vi "AlliGator Filter Phasors in ROI(s).vi"(7 "Phasor Plot Image":T1, 8 "error in (no error)":errorcluster, 9 "All Phasor Plot ROIs":bool, 10 "Selected Phasor Plot ROI(s)":bool, 11 "Phasor Array in":csg[](array[numeric])) -> (0 "error out":errorcluster, 1 "Message":string, 3 "Phasor Array out":csg[](array[numeric]))   [LabVIEW 2021, in "AlliGator Phasor Plot.lvlib"]
doc: "Returns an array of phasor values located within the selected Phasor Plot ROI (or All ROIs)."
uses:
  AlliGator Phasor Plot.lvlib
  <vilib>/vision/Image Controls.llb/IMAQ Image.ctl
  Globals, Variables, Constants/AlliGator Variables List.ctl
  Phasor Ratio/AlliGator Phasor Plot Reference Points.ctl
  91eb7ac0-7abc-46e1-b76d-bce32f8ebfb4.vi
  <userlib>/_OpenG.lib/array/array.llb/Filter 1D Array (CSG)__ogtk.vi
  ROIs/AlliGator ROIs.lvlib
  <vilib>/vision/NI_Vision_Development_Module.lvlib
  Globals, Variables, Constants/AlliGator Globals, Variables & Constants.lvlib
  Phasor Ratio/AlliGator Phasor Ratio.lvlib
  Strings/Strings.lvlib
  <userlib>/_OpenG.lib/array/array.llb/openg_array.lvlib
  Error/Error.lvlib
panel:
  # "see the AlliGator License on the block diagram (Ctrl+E or Window:Show Block Diagram)"
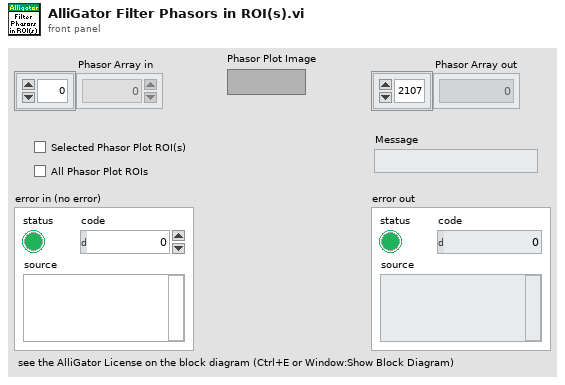
[diagram p1: front panel]
types:
  T1 = typedef "IMAQ Image.ctl" = refnum<image>
  T2 = typedef "AlliGator Phasor Ratio.lvlib/AlliGator Phasor Plot Reference Points.ctl" = cluster{"O_h":dbl, "O_v":dbl, "1_h":dbl, "1_v":dbl}
  T3 = typedef "AlliGator Globals, Variables & Constants.lvlib/AlliGator Variables List.ctl" = enum16{"---- GUI ----", "GUI:Initialization Status", "GUI:State Indicators Refnum", "GUI:Original AlliGator Menu Items", "GUI:Current Action Loop State", "GUI:Script in progress", "GUI:Playback", "GUI:Loop Playback", "GUI:Search ROI Used", "GUI:Search ROI", "Decay Graph Max Legend Size", "Intensity Graph Max Legend Size", "Decay Statistics Graph Max Legend Size", "Phasor Graph Max Legend Size", "Phasor Ratio Graph Max Legend Size", "Lifetime Graph Max Legend Size", "---- Files ----", "Files:Export Dataset Frames as Individual Files", "Files:Show Batch Export Help Balloons", "Files:Frames in Dataset", "Files:ptu File Frame Start Indices", "Files:Current Frame in Dataset", "Files:Current Frame Timestamp", "Files:Dataset Loaded", "Files:Dataset Metadata", "Files:Dataset Channel", "Files:Dataset Data Description", "Files:Background Dataset Metadata", "Files:Background Dataset Channel", "Files:Background Dataset Data Description", "Files:Background File Subtraction", "Files:Background File Path", "Files:Background File Pile-up Correction", "Files:Background File Pixel Well Capacity", "Files:Background File Scaling Factor", "Files:Current Dataset Load Settings", "Files:Dataset Path", "Files:ICCD-specific Information", "Files:Macrotime Gate Separation", "------ Python Plugins ------", "Python Plugins:Information", "Python Plugins:Python Session", "Python Plugins:Valid Python Session?", "---- Source Image ----", "Source Image:ROIs", "Source Image:Current ROI", "Source Image:ROI Event Refnum", "X_Source Image:Display Range", "X_Source Image:Palette Information", "X_Source Image:Type of Displayed Image", "X_Time Gate Slider", "Source Image:Palette List", "Source Image:Scale", "Source Image:ROI Overlay Color", "Source Image:Overlay to Erase", "Source Image:Is Displayed Image Accumulated", "Source Image:White Light Image Modified", "Source Image:Mask Image Modified", "---- Image Profile Window ----", "Image Profile:Window Event Refnum", "Image Profile:IntensityType", "Image Profile:Intensity Average Type", "Image Profile:Intensity-weighted SDV", "Image Profile:Box Profile Type", "Image Profile:Window Open", "Image Profile:Plotted Fit Parameter", "------ Phasor Graph -------", "Phasor Graph:Show Line", "---- Phasor Plot ---", "Phasor Plot:Parameters Changed", "Phasor Plot:FLI Dataset Modified since last Calculation", "Phasor Harmonics Data", "Selected Phasor Harmonics", "Phasor Harmonic Manager Event Refnum", "Phasor Plot:ROIs", "Phasor Plot:Current ROI", "Phasor Plot:ROI Event Refnum", "Phasor Plot:Image Reference Points", "Phasor Plot:Computed", "Phasor Plot:Palette Information", "Phasor Plot:Palette List", "Phasor Plot:Phasor Ratio Palette Information", "Phasor Plot:Phasor Ratio Palette List", "Phasor Plot:Image Scale", "Phasor Plot:Image Overlay to Erase", "Phasor Plot:Image Elements to Update", "Phasor Plot:Current Calculation Parameters", "Phasor Plot:Current Calibration Options", "Phasor Plot:Reset Cumulated Phasor Plot", "Phasor Plot:Reference 1", "Phasor Plot:Lifetime Reference 1", "Phasor Plot:Reference 1 Frequency", "Phasor Plot:Reference 2", "Phasor Plot:Lifetime Reference 2", "Phasor Plot:Reference 2 Frequency", "---- Decay Analysis ----", "Number of Selected Decays to Fit", "LS Fit Results", "LAR Fit Results", "BS Fit Results", "Last Decay Max - Min", "Best Fit Parameters", "Best Fit Parameter Names", "Actual Size X", "Actual Size Y", "Binning X", "Binning Y", "Actual # Gates", "Dataset Number", "Gates to...", "Gates Skipped", "Gates to keep", "Gate Step", "Gate Separation", "Reversed Gates", "Pile-up Correction", "Pixel Well Capacity", "Background Subtracted", "Background Subtraction Method", "Background Definition Range", "Background File (deprecated)", "Number of Dataset Accumulated", "Array of Accumulated Dataset Paths", "Do Averaged Datasets", "Destination File Path", "Process Plot Target", "Use 1/D as Phasor Frequency", "---- Decay Fit Parameter Map -----", "Decay Fit Parameter Map:Palette Information", "Decay Fit Parameter Map:Palette List", "Decay Fit Parameter Map:X Resolution", "Decay Fit Parameter Map:Y Resolution", "---- Parameter Map ----", "Parameter Map:Palette Information", "Parameter Map:Palette List", "------- Local Decay Window ---------", "Local Decay Graph Window:Event Refnum", "Local Decay Graph Window:Use normalized IRF for convolution", "----- Miscellaneous ----", "Misc:Skippable Dialog Windows Status"}
  T4 = typedef "Image Type" = u32
  T5 = typedef "Image.lvlib/Named ROI Description.ctl" = cluster{"ROI Descriptor":T6, "ROI Name":string, "Overlay Color":u32}
  T6 = typedef "ROI Descriptor" = cluster{"Global Rectangle":i32[], "Contours":cluster{"ID":enum32{"External", "Internal"}, "Type":u32, "Coordinates":i32[]}[]}
  T7 = cluster{"Phasor Plot x":dbl, "Phasor Plot y":dbl}
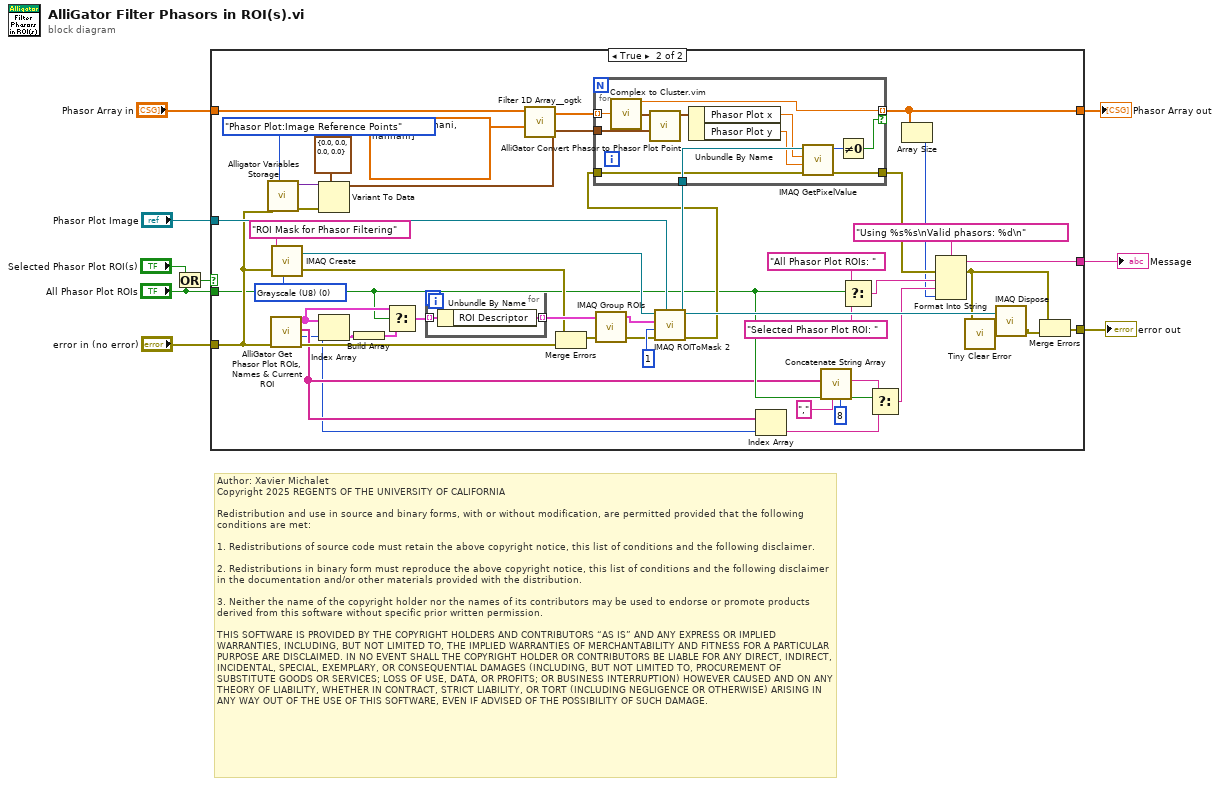
[diagram p0: block diagram]
diagram:
  # "Author: Xavier Michalet\nCopyright 2025 REGENTS OF THE UNIVERSITY OF CALIFORNIA\n\nRedistribution and use in source and binary forms, with or without modification, are permitted provided that the following conditions are met:\n\n1. Redistributions of source code must retain the above copyright notice, this list of conditions and the following disclaimer.\n\n2. Redistributions in binary form must reproduce the above copyright notice, this list of conditions and the following disclaimer in the documentation and/or other materials provided with the distribution.\n\n3. Neither the name of the copyright holder nor the names of its contributors may be used to endorse or promote products derived from this software without specific prior written permission.\n\nTHIS SOFTWARE IS PROVIDED BY THE COPYRIGHT HOLDERS AND CONTRIBUTORS “AS IS” AND ANY EXPRESS OR IMPLIED WARRANTIES, INCLUDING, BUT NOT LIMITED TO, THE IMPLIED WARRANTIES OF MERCHANTABILITY AND FITNESS FOR A PARTICULAR PURPOSE ARE DISCLAIMED. IN NO EVENT SHALL THE COPYRIGHT HOLDER OR CONTRIBUTORS BE LIABLE FOR ANY DIRECT, INDIRECT, INCIDENTAL, SPECIAL, EXEMPLARY, OR CONSEQUENTIAL DAMAGES (INCLUDING, BUT NOT LIMITED TO, PROCUREMENT OF SUBSTITUTE GOODS OR SERVICES; LOSS OF USE, DATA, OR PROFITS; OR BUSINESS INTERRUPTION) HOWEVER CAUSED AND ON ANY THEORY OF LIABILITY, WHETHER IN CONTRACT, STRICT LIABILITY, OR TORT (INCLUDING NEGLIGENCE OR OTHERWISE) ARISING IN ANY WAY OUT OF THE USE OF THIS SOFTWARE, EVEN IF ADVISED OF THE POSSIBILITY OF SUCH DAMAGE."
  n1 = Or(x="Selected Phasor Plot ROI(s)", y="All Phasor Plot ROIs") -> (x .or. y?=w6:bool)
  n2 = case shown="True" w6 {
    tunnel: "error in (no error)" -> [w10 w38]
    tunnel: "All Phasor Plot ROIs" -> [_ w22]
    tunnel: "Phasor Array in" -> [w11 w37]
    tunnel: [w11 w17] -> w4
    tunnel: [w10 w13] -> w3
    tunnel: "Phasor Plot Image" -> [_ w44]
    tunnel: [_ w31] -> w1
    frame False {
    }
    frame True {
      w56 = T4 0 items=["Grayscale (U8)", "Grayscale (I16)", "Grayscale (SGL)", "Complex (CSG)", "RGB (U32)", "HSL (U32)", "RGB (U64)", "Grayscale (U16)"] ("Image Type")
      n3 = call "Alligator Variables Storage.vi"("AlliGator Variable"=AlliGator_Variables_List."Phasor Plot:Image Reference Points" ("Alligator Variable"), "Error In"=w38) -> ("Error Out"=w40:errorcluster, "Data out"=w41:variant)  [unwired: 7 in, 1 out]
      n4 = call "AlliGator Get Phasor Plot ROIs, Names & Current ROI.vi"("Error In"=w38) -> ("Error Out"=w48:errorcluster, "Current ROI"=w20:i32, "ROI Names"=w21:string[], "Stored ROIs"=w51:T5[])  [unwired: 7 in]
      n5 = call "IMAQ Create"("Image Name"="ROI Mask for Phasor Filtering", "Image Type"=w56, "error in (no error)"=w38) -> ("New Image"=w45:T1, "error out"=w46:errorcluster)  [unwired: 2 in]
      n6 = Variant To Data(error in=w40, type=T2 {"O_h"=0.0, "O_v"=0.0, "1_h"=0.0, "1_v"=0.0} ("Phasor Plot Reference Points"), Variant=w41) -> (data=w35:T2)  [unwired: 1 out]
      n7 = Index Array(array=w51, index=w20) -> (element=w55:T5)
      n8 = Build Array(w55) -> (w54:T5[])
      n9 = Select(t=w51, s=w22, f=w54) -> (s? t:f=w50:T5[])
      n10 = for {
        tunnel: w50 -> [w70] mode=indexing
        tunnel: [w69] -> w49 mode=indexing
        n11 = Unbundle By Name(w70) -> ("ROI Descriptor"=w69:T6)
      }
      n12 = call-poly <userlib>:"Filter 1D Array__ogtk.vi"("items to filter"=csg[] [nan+0.0i, 0.0+nani, nan+nani] ("Element(s) to Remove"), "array"=w37) -> ("filtered array"=w34:csg[])  [unwired: 4 in, 1 out]
      n13 = Merge Errors(w46, w48) -> (w47:errorcluster)
      n14 = call "IMAQ Group ROIs"("error in (no error)"=w47, "ROI Descriptors"=w49) -> ("error out"=w52:errorcluster, "ROI Descriptor out"=w43:T6)  [unwired: 2 in]
      n15 = call "IMAQ ROIToMask 2"("Image Model"=w44, "error in (no error)"=w52, "Filling Value (255)"=1, "ROI Descriptor"=w43, "Image"=w45) -> ("error out"=w32:errorcluster, "Image Out"=w33:T1)  [unwired: 4 in, 1 out]
      n16 = for {
        tunnel: w35 -> [w68]
        tunnel: w34 -> [w66] mode=indexing
        tunnel: [w66] -> w17 mode=indexing if=w59
        tunnel: w33 -> [w65]
        tunnel: w32 -> [w61]
        tunnel: [w58] -> w30
        n17 = call "Complex to Cluster.vim"("x + iy"=w66) -> ("Complex Coordinates"=w67:cluster{sgl, sgl})  [unwired: 8 in]
        n18 = call "AlliGator Convert Phasor to Phasor Plot Point.vi"("Phasor Plot Reference Points"=w68, "Phasor"=w67) -> ("Phasor Plot Point"=w64:T7)  [unwired: 9 in]
        n19 = Unbundle By Name(w64) -> ("Phasor Plot x"=w63:dbl, "Phasor Plot y"=w62:dbl)
        n20 = call "IMAQ GetPixelValue"("Image"=w65, "X Coordinate"=w63, "Y Coordinate"=w62, "error in (no error)"=w61) -> ("Pixel Value (U8)"=w60:u8, "error out"=w58:errorcluster)  [unwired: 2 in, 3 out]
        n21 = Not Equal To 0?(x=w60) -> (x != 0?=w59:bool)
      }
      n22 = Index Array(array=w21, index=w20) -> (element=w19:string)
      n23 = call "Concatenate String Array.vi"("Max Number of Elements (None: -1)"=8, "Separator (TAB)"=",", "String Array"=w21) -> ("Formatted String"=w23:string)  [unwired: 8 in]
      n24 = Select(t="All Phasor Plot ROIs: " ("format string"), s=w22, f="Selected Phasor Plot ROI: " ("format string")) -> (s? t:f=w26:string)
      n25 = Select(t=w23, s=w22, f=w19) -> (s? t:f=w18:string)
      n26 = Array Size(array=w17) -> (size(s)=w16:i32)
      n27 = Format Into String(format string="Using %s%s\nValid phasors: %d\n", error in=w30, w26, w18, w16) -> (resulting string=w31:string, error out=w14:errorcluster)  [unwired: 1 in]
      n28 = call "Tiny Clear Error.vi"("Error In"=w14) -> ("no Error Out"=w12:errorcluster)  [unwired: 8 in]
      n29 = call "IMAQ Dispose"("Image"=w33, "error in (no error)"=w12) -> ("error out"=w15:errorcluster)  [unwired: 4 in]
      n30 = Merge Errors(w14, w15) -> (w13:errorcluster)
    }
  }
  "Phasor Array out" <- w4
  "error out" <- w3
  "Message" <- w1
